vi "Bool.vi"(4 "Boolean":bool) -> (1 "Abs_Boolean.lvclass":refnum<class "Abs_Boolean.lvclass">)   [LabVIEW 2021, in "Const_Bool.lvclass"]
uses:
  Const_Bool.lvclass
  Abs_Types/Boolean/Abs_Boolean.lvclass
  C:/Program Files (x86)/National Instruments/LabVIEW 2021/vi.lib/TSA/Abstract Data Classes/Abs_Types/Boolean/Abs_Boolean.lvclass
  Const_Bool.lvclass/Const_Bool.ctl
  Properties/Write Value.vi
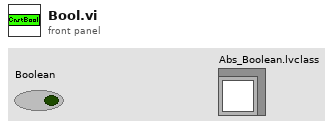
[diagram p1: front panel]
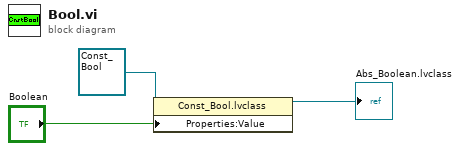
[diagram p0: block diagram]
diagram:
  n1 = property class="Const_Bool.lvclass"(reference=refnum<class "Const_Bool.lvclass"> refnum ("Constants.lvlib:Boolean.lvclass"), "Properties:Value"="Boolean") -> (reference out=→"Abs_Boolean.lvclass":refnum<class "Const_Bool.lvclass">)  [unwired: 1 in, 1 out]
